vi "Main - Write Waveform to FPGA.vi"(11 "Total Waveform data points":u32) -> (1 "All points written?":bool, 2 "Element address final":u32, 3 "Waveform data points written final":u32)   [LabVIEW 2015]
uses:
  <vilib>/Platform/TimedLoop/XDataNode/timing_clust.ctl
  <vilib>/Platform/TimedLoop/XDataNode/nitl_modes.ctl
  <vilib>/Platform/TimedLoop/XDataNode/wakeup.ctl
  Output Waveform and drive Galvo/DRAM data index.ctl
  <vilib>/rvi/Emulation/niFpgaSctlEmulationGetInTimedLoop.vi
  <vilib>/rvi/Emulation/niFpgaEmulationReportErrorSimple.vi
  <vilib>/rvi/Emulation/niFpgaGetClockAttributes.vi
  <vilib>/rvi/Emulation/niFpgaCriticalErrorInLSC.vi
  <vilib>/Platform/TimedLoop/XDataNode/XDataNode.xnode
  <vilib>/Platform/TimedLoop/XDataNode/XDNodeRunTimeDep.lvlib
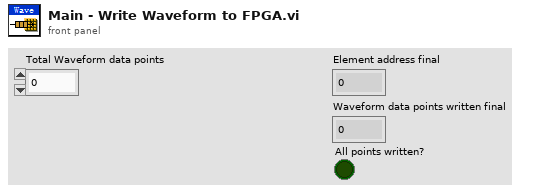
[diagram p1: front panel]
types:
  T1 = cluster{"Numeric 1":u32, "Numeric 2":u32, "Numeric 3":u32, "Numeric 4":u32, "Numeric 5":u32, "Numeric 6":u32, "Numeric 7":u32, "Numeric 8":u32, "Numeric 9":u32, "Numeric 10":u32, "Numeric 11":u32, "Numeric 12":u32, "Numeric 13":u32, "Numeric 14":u32, "Numeric 15":u32, "Numeric 16":u32}
  T2 = typedef "DRAM data index.ctl" = enum16{"Numeric 1", "Numeric 2", "Numeric 3", "Numeric 4", "Numeric 5", "Numeric 6", "Numeric 7", "Numeric 8", "Numeric 9", "Numeric 10", "Numeric 11", "Numeric 12", "Numeric 13", "Numeric 14", "Numeric 15", "Numeric 16"}
  T3 = typedef "XDNodeRunTimeDep.lvlib/timing_clust.ctl" = cluster{"Expected End [f-1]":u64, "Actual End [f-1]":u64, "Finished Late? [f-1]":bool, "Expected End [i-1]":u64, "Actual End [i-1]":u64, "Finished Late? [i-1]":bool, "Expected Start [i]":u64, "Actual Start [i]":u64, "Expected Start [f]":u64, "Actual Start [f]":u64, "Source Name":string, "Structure Name":string, "Period":i64, "Deadline":i64, "Offset":i64, "Start":i64, "Priority":i32, "Timeout":i32, "Mode":T4, "Wakeup Reason":T5, "Error":errorcluster, "Source Type":string, "Secondary Source Type":string, "Global End Time":u64, "Global Start Time":u64, "Frame Duration":u64, "Iteration Duration":u64, "Assigned CPU":i32, "I/O Scan Engine Mode":u32}
  T4 = typedef "XDNodeRunTimeDep.lvlib/nitl_modes.ctl" = enum32{"No Change", "Process missed periods, maintain original phase", "Discard missed periods, maintain original phase", "Process missed periods, ignore original phase", "Discard missed periods, ignore original phase"}
  T5 = typedef "XDNodeRunTimeDep.lvlib/wakeup.ctl" = enum32{"Normal", "Aborted", "Asynchronous wakeup", "Timing source error", "Timed loop error", "Timeout"}
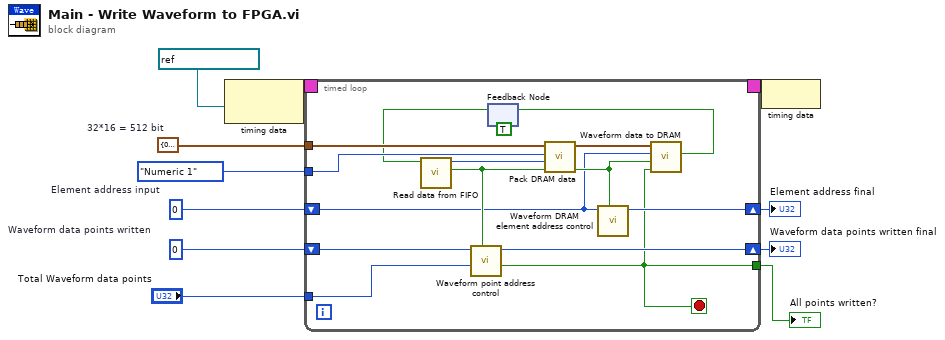
[diagram p0: block diagram]
diagram:
  w8 = T1 {"Numeric 1"=0, "Numeric 2"=0, "Numeric 3"=0, "Numeric 4"=0, "Numeric 5"=0, "Numeric 6"=0, "Numeric 7"=0, "Numeric 8"=0, "Numeric 9"=0, "Numeric 10"=0, "Numeric 11"=0, "Numeric 12"=0, "Numeric 13"=0, "Numeric 14"=0, "Numeric 15"=0, "Numeric 16"=0}  # 32*16 = 512 bit
  w4 = u32 0  # Element address input
  w5 = u32 0  # Waveform data points written
  n1 = node-c288(refnum<k21> "DRAM Clock" ("源名称")) -> (w11:T3)
  n2 = timed-loop {
    timing: w11 -> [_]
    timing-out: [_] -> w10
    tunnel: w8 -> [w25]
    tunnel: DRAM_data_index."Numeric 1" ("DRAM Index in") -> [w24]
    tunnel: "Total Waveform data points" -> [w22]
    tunnel: [w15] -> w1
    shift-right: [w20] -> w2
    shift-left: w5 -> [w19]
    shift-right: [w17] -> w3
    shift-left: w4 -> [w16]
    stop <- w15 stop-if-true
    n3 = feedback #1(TRUE ("Input ready")) -> (w13:bool)
    n4 = call "Read data from FIFO.vi"("Ready for Input"=w13) -> ("Output Valid"=w21:bool, "Data"=w26:u32)  [unwired: 9 in]
    n5 = call "Waveform point address control.vi"("Input Valid"=w21, "Total elements"=w22, "Elements wrote in"=w19) -> ("All points written"=w15:bool, "Elements wrote out"=w20:u32)  [unwired: 4 in]
    n6 = call "Pack DRAM data.vi"("input valid?"=w21, "data to be packed"=w26, "DRAM Index in"=w24, "packer in"=w25) -> ("output valid?"=w18:bool, "packer out"=w23:T1)  [unwired: 5 in, 1 out]
    n7 = call "Waveform DRAM element address control.vi"("DRAM address input in"=w16, "output valid?"=w18) -> ("DRAM address output"=w17:u32)  [unwired: 8 in]
    n8 = call "Waveform data to DRAM.vi"("packer out"=w23, "Element address input"=w16, "Package input valid?"=w18, "All points written?"=w15) -> ("Input ready"=w14:bool)  [unwired: 6 in]
    n9 = feedback-in #1(w14) -> ()
  }
  "Element address final" <- w3
  "Waveform data points written final" <- w2
  "All points written?" <- w1
  n10 = node-c288(w10) -> ()
